vi "B_Globals.vi"() -> ()   [LabVIEW 2019]
panel:
  out "G_B_set[T]":dbl
  out "Rem_stable_B":bool
  out "Remote_Go":bool
  in  "Remote_Rate":dbl
  out "Remote_run":bool
  in  "Remote_set":dbl
  out "B [T]":dbl
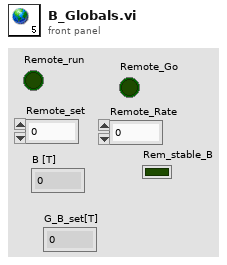
[diagram p1: front panel]
diagram:
